vi "DefaultSourceTag.vi"(8 "error in (no error)":errorcluster, 11 "OriginVI":string) -> (0 "error out":errorcluster, 3 "SourceTag":string)   [LabVIEW 2026, in "Lumberjack.lvlib"]
doc: "Pure default-tag derivation. From the emitting VI name, take the base name (drop path and .vi), then Sanitize it to a single node, used when the caller supplies no sourceTag (SRS-LMBR-013, 017). No state, no I/O; deterministic."
uses:
  Lumberjack.lvlib
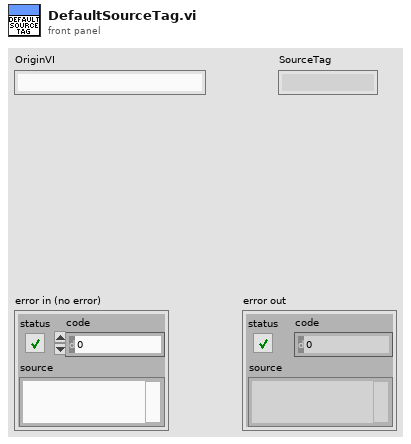
[diagram p1: front panel]
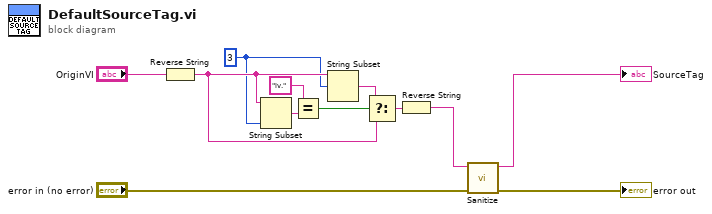
[diagram p0: block diagram]
diagram:
  w2 = 3 ("length (rest)")
  n1 = Reverse String(1:"OriginVI") -> (0:w3:string)
  n2 = String Subset(string=w3, length (rest)=w2) -> (substring=w8:string)  [unwired: 1 in]
  n3 = Equal?(x="iv." ("search string/char (-)"), y=w8) -> (x = y?=w9:bool)
  n4 = String Subset(string=w3, offset (0)=w2) -> (substring=w1:string)  [unwired: 1 in]
  n5 = Select(t=w1, s=w9, f=w3) -> (s? t:f=w5:string)
  n6 = Reverse String(1:w5) -> (0:w4:string)
  n7 = call "Sanitize.vi"("error in (no error)"="error in (no error)", "RawTag"=w4) -> ("error out"=→"error out":errorcluster, "CleanTag"=→"SourceTag":string)  [unwired: 8 in]
